vi "SimpleDevStatus.vi"(7 "error in":errorcluster, 9 "ON/OFF":bool, 10 "VISA resource name in":refnum<visa-resource-name>) -> (0 "error out":errorcluster, 2 "Device Status":T1, 3 "VISA resource name out":refnum<visa-resource-name>)   [LabVIEW 2014]
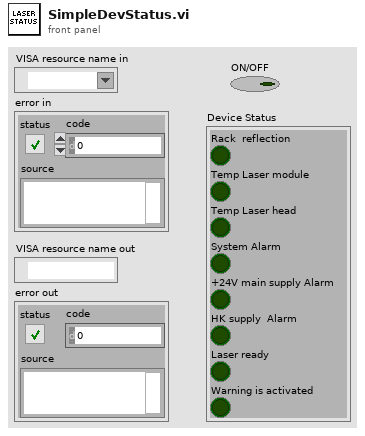
[diagram p1: front panel]
types:
  T1 = cluster{"Rack  reflection":bool, "Temp Laser module":bool, "Temp Laser head":bool, "System Alarm":bool, "+24V main supply Alarm":bool, "HK supply  Alarm":bool, "Laser ready":bool, "Warning is activated":bool}
  T2 = cluster{"Boolean array[0]":bool, "Boolean array[1]":bool, "Boolean array[2]":bool, "Boolean array[3]":bool, "Boolean array[4]":bool, "Boolean array[5]":bool, "Boolean array[6]":bool, "Boolean array[7]":bool}
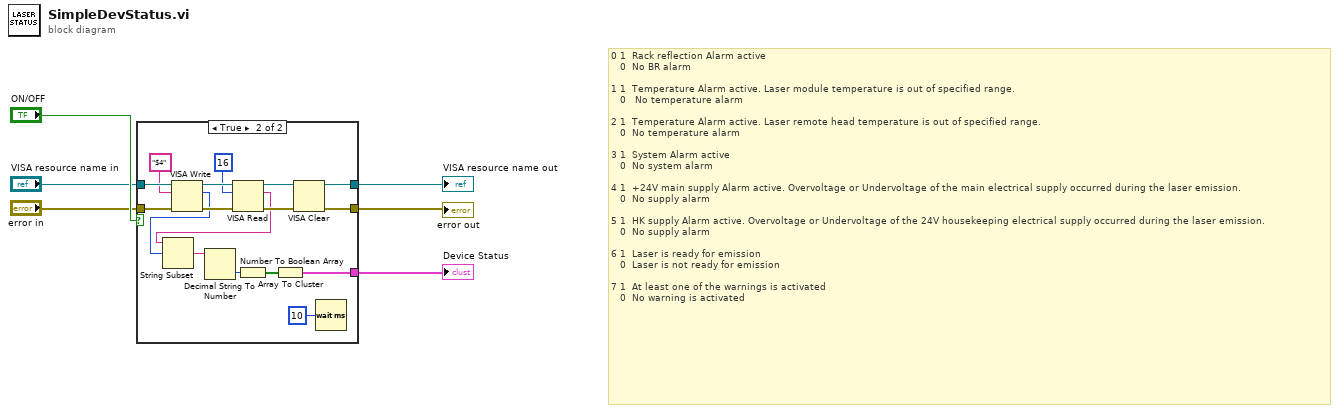
[diagram p0: block diagram]
diagram:
  # "0 1  Rack reflection Alarm active\n   0  No BR alarm\n\n1 1  Temperature Alarm active. Laser module temperature is out of specified range.\n   0   No temperature alarm\n\n2 1  Temperature Alarm active. Laser remote head temperature is out of specified range.\n   0  No temperature alarm\n\n3 1  System Alarm active\n   0  No system alarm\n\n4 1  +24V main supply Alarm active. Overvoltage or Undervoltage of the main electrical supply occurred during the laser emission.\n   0  No supply alarm\n\n5 1  HK supply Alarm active. Overvoltage or Undervoltage of the 24V housekeeping electrical supply occurred during the laser emission.\n   0  No supply alarm\n\n6 1  Laser is ready for emission\n   0  Laser is not ready for emission\n\n7 1  At least one of the warnings is activated\n   0  No warning is activated"
  n1 = case shown="True" "ON/OFF" {
    tunnel: "VISA resource name in" -> [w8 w23]
    tunnel: "error in" -> [w7 w22]
    tunnel: [w8 w18] -> w3
    tunnel: [w7 w17] -> w2
    tunnel: [_ w9] -> w1
    frame False {
    }
    frame True {
      n2 = VISA Write(VISA resource name=w23, write buffer="$4", error in (no error)=w22) -> (VISA resource name out=w24:refnum<visa-resource-name>, return count=w10:u32, error out=w25:errorcluster)
      n3 = VISA Read(VISA resource name=w24, byte count=u32 16, error in (no error)=w25) -> (VISA resource name out=w20:refnum<visa-resource-name>, read buffer=w11:string, error out=w19:errorcluster)  [unwired: 1 out]
      n4 = String Subset(string=w11, offset (0)=w10) -> (substring=w12:string)  [unwired: 1 in]
      n5 = Decimal String To Number(string=w12) -> (number=w13:i32)  [unwired: 2 in, 1 out]
      n6 = Number To Boolean Array(number=w13) -> (Boolean array=w14:bool[])
      n7 = Array To Cluster(array=w14) -> (cluster=w9:T2)
      n8 = VISA Clear(VISA resource name=w20, error in (no error)=w19) -> (VISA resource name out=w18:refnum<visa-resource-name>, error out=w17:errorcluster)
      n9 = Wait (ms)(milliseconds to wait=u32 10) -> ()  [unwired: 1 out]
    }
  }
  "Device Status" <- w1
  "VISA resource name out" <- w3
  "error out" <- w2
